vi "2BALL1~1.VI"(1 "Run?":bool) -> (0 "Done?":bool)   [LabVIEW 2013]
uses:
  Globals/Homes.vi
  Globals/Useful Values.vi
panel:
  out "Time Elapsed":dbl
  out "Sum":dbl
  out "Ready for Vision?":bool
  out "Side":dbl
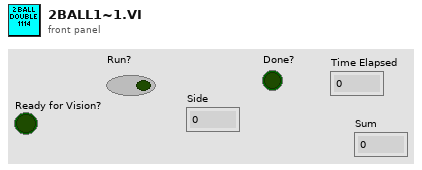
[diagram p1: front panel]
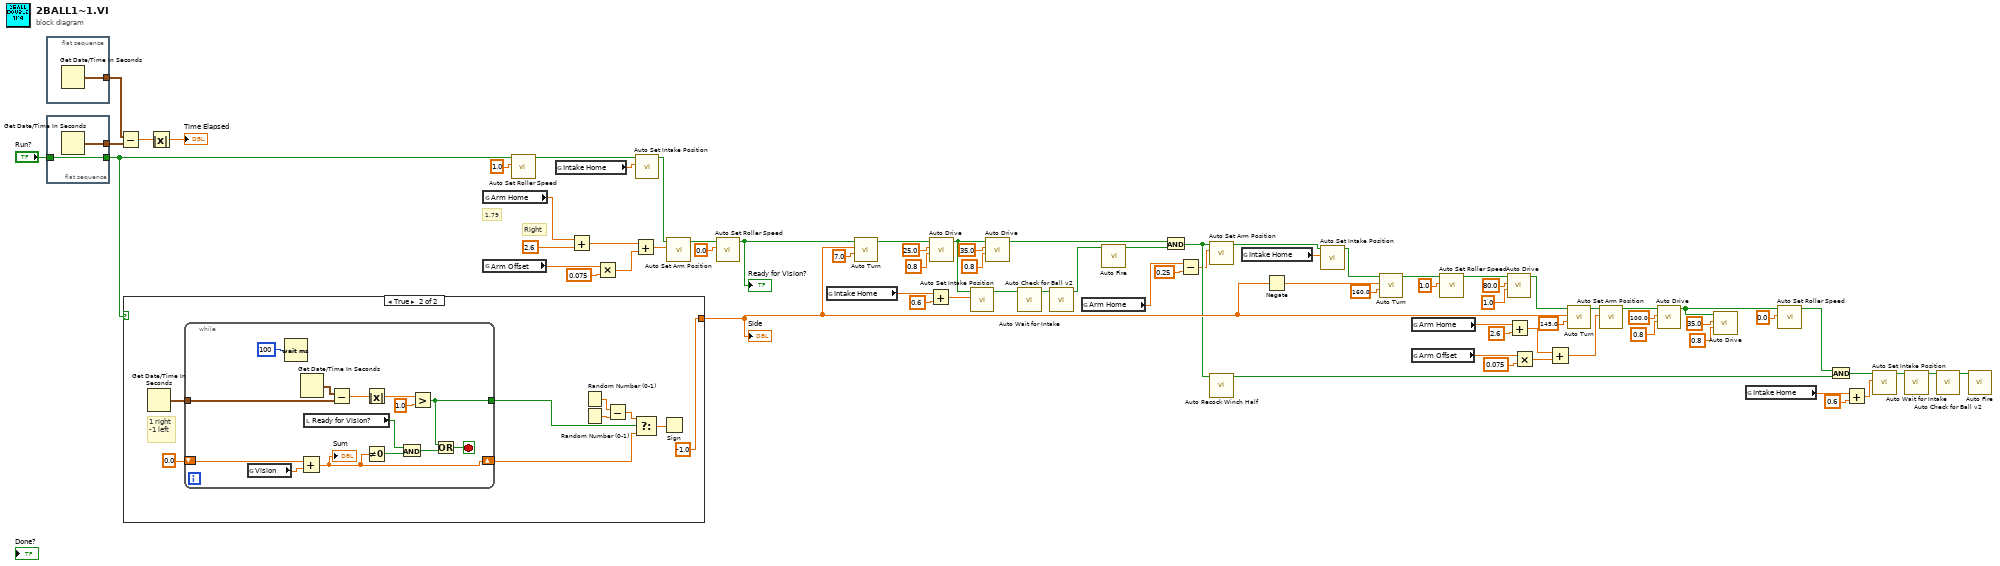
[diagram p0: block diagram]
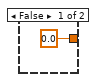
[diagram p2: hidden frame]
diagram:
  # "Right"
  # "1.79"
  n1 = flat-sequence {
    tunnel: [w77] -> w64
    frame #0 {
      n2 = Get Date/Time In Seconds() -> (seconds since 1Jan1904=w77:timestamp)
    }
  }
  n3 = flat-sequence {
    tunnel: "Run?" -> [w79]
    tunnel: [w79] -> w65
    tunnel: [w78] -> w61
    frame #0 {
      n4 = Get Date/Time In Seconds() -> (seconds since 1Jan1904=w78:timestamp)
    }
  }
  n5 = Subtract(x=w64, y=w61) -> (x-y=w63:dbl)
  n6 = case shown="True" w65 {
    tunnel: [0.0 -1.0] -> w56
    frame False {
    }
    frame True {
      # "1 right\n-1 left"
      n7 = Get Date/Time In Seconds() -> (seconds since 1Jan1904=w88:timestamp)
      n8 = while {
        shift-right: [w99] -> w83
        shift-left: 0.0 -> [w102]
        tunnel: w88 -> [w97]
        tunnel: [w90] -> w84
        stop <- w92 stop-if-true
        n9 = global read "Useful Values.vi" "Vision"() -> (w103:dbl)
        n10 = Wait (ms)(milliseconds to wait=u32 100) -> ()  [unwired: 1 out]
        n11 = Add(x=w102, y=w103) -> (x+y=w99:dbl)
        "Sum" <- w99
        n12 = Get Date/Time In Seconds() -> (seconds since 1Jan1904=w96:timestamp)
        n13 = local read "Ready for Vision?"() -> (w100:bool)
        n14 = Subtract(x=w96, y=w97) -> (x-y=w95:dbl)
        n15 = Absolute Value(x=w95) -> (abs(x)=w94:dbl)
        n16 = Not Equal To 0?(x=w99) -> (x != 0?=w98:bool)
        n17 = And(x=w100, y=w98) -> (x .and. y?=w91:bool)
        n18 = Greater?(x=w94, y=1.0) -> (0:w90:bool)
        n19 = Or(x=w90, y=w91) -> (x .or. y?=w92:bool)
      }
      n20 = Random Number (0-1)() -> (number: 0 to 1=w85:dbl)
      n21 = Random Number (0-1)() -> (number: 0 to 1=w86:dbl)
      n22 = Subtract(x=w85, y=w86) -> (x-y=w87:dbl)
      n23 = Select(t=w87, s=w84, f=w83) -> (s? t:f=w82:dbl)
      n24 = Sign(1:w82) -> ()  [unwired: 1 out]
    }
  }
  "Side" <- w56
  n25 = Absolute Value(x=w63) -> (abs(x)=→"Time Elapsed":dbl)
  n26 = global read "Homes.vi" "Arm Home"() -> (w75:dbl)
  n27 = global read "Useful Values.vi" "Arm Offset"() -> (w73:dbl)
  n28 = call "Auto Set Roller Speed.vi"("Value"=1.0, "Run?"=w65) -> ("Done"=w68:bool)  [unwired: 9 in]
  n29 = global read "Homes.vi" "Intake Home"() -> (w76:dbl)
  n30 = Add(x=w75, y=2.6) -> (x+y=w70:dbl)
  n31 = Multiply(x=w73, y=0.075) -> (x*y=w71:dbl)
  n32 = Add(x=w70, y=w71) -> (x+y=w59:dbl)
  n33 = call "Auto Set Intake Position.vi"("Intake Position"=w76, "Run?"=w68) -> ("Done"=w60:bool)  [unwired: 9 in]
  n34 = call "Auto Set Arm Position.vi"("Arm Position"=w59, "Run?"=w60) -> ("Done"=w58:bool)  [unwired: 9 in]
  n35 = call "Auto Set Roller Speed.vi"("Value"=0.0, "Run?"=w58) -> ("Done"=w57:bool)  [unwired: 9 in]
  "Ready for Vision?" <- w57
  n36 = global read "Homes.vi" "Intake Home"() -> (w50:dbl)
  n37 = call "Auto Turn.vi"("Turn Amount"=7.0, "+/-?"=w56, "Run?"=w57) -> ("Done"=w47:bool)  [unwired: 8 in]
  n38 = Add(x=w50, y=0.6) -> (x+y=w48:dbl)
  n39 = call "Auto Drive.vi"("Speed"=0.8, "Amount"=25.0, "Run?"=w47) -> ("Done"=w41:bool)  [unwired: 8 in]
  n40 = call "Auto Set Intake Position.vi"("Intake Position"=w48, "Run?"=w41) -> ("Done"=w46:bool)  [unwired: 9 in]
  n41 = call "Auto Drive.vi"("Speed"=0.8, "Amount"=35.0, "Run?"=w41) -> ("Done"=w44:bool)  [unwired: 8 in]
  n42 = call "Auto Wait for Intake.vi"("Run?"=w46) -> ("Done"=w43:bool)  [unwired: 10 in]
  n43 = call "Auto Check for Ball v2.vi"("Run?"=w43) -> ("Done"=w42:bool)  [unwired: 10 in]
  n44 = global read "Homes.vi" "Arm Home"() -> (w34:dbl)
  n45 = call "Auto Fire.vi"("Run?"=w42) -> ("Done"=w45:bool)  [unwired: 10 in]
  n46 = And(x=w44, y=w45) -> (x .and. y?=w35:bool)
  n47 = Subtract(x=w34, y=0.25) -> (x-y=w32:dbl)
  n48 = call "Auto Set Arm Position.vi"("Arm Position"=w32, "Run?"=w35) -> ("Done"=w31:bool)  [unwired: 9 in]
  n49 = call "Auto Recock Winch Half.vi"("Run?"=w35) -> ("Done"=w12:bool)  [unwired: 10 in]
  n50 = global read "Homes.vi" "Intake Home"() -> (w29:dbl)
  n51 = Negate(x=w56) -> (-x=w5:dbl)
  n52 = call "Auto Set Intake Position.vi"("Intake Position"=w29, "Run?"=w31) -> ("Done"=w30:bool)  [unwired: 9 in]
  n53 = call "Auto Turn.vi"("Turn Amount"=160.0, "+/-?"=w5, "Run?"=w30) -> ("Done"=w37:bool)  [unwired: 8 in]
  n54 = global read "Homes.vi" "Arm Home"() -> (w21:dbl)
  n55 = global read "Useful Values.vi" "Arm Offset"() -> (w25:dbl)
  n56 = call "Auto Set Roller Speed.vi"("Value"=1.0, "Run?"=w37) -> ("Done"=w38:bool)  [unwired: 9 in]
  n57 = call "Auto Drive.vi"("Speed"=1.0, "Amount"=80.0, "Run?"=w38) -> ("Done"=w19:bool)  [unwired: 8 in]
  n58 = Add(x=w21, y=2.6) -> (x+y=w22:dbl)
  n59 = Multiply(x=w25, y=0.075) -> (x*y=w23:dbl)
  n60 = Add(x=w22, y=w23) -> (x+y=w20:dbl)
  n61 = call "Auto Turn.vi"("Turn Amount"=145.0, "+/-?"=w56, "Run?"=w19) -> ("Done"=w18:bool)  [unwired: 8 in]
  n62 = call "Auto Set Arm Position.vi"("Arm Position"=w20, "Run?"=w18) -> ("Done"=w1:bool)  [unwired: 9 in]
  n63 = call "Auto Drive.vi"("Speed"=0.8, "Amount"=100.0, "Run?"=w1) -> ("Done"=w3:bool)  [unwired: 8 in]
  n64 = call "Auto Drive.vi"("Speed"=0.8, "Amount"=35.0, "Run?"=w3) -> ()  [unwired: 8 in, 1 out]
  n65 = global read "Homes.vi" "Intake Home"() -> (w8:dbl)
  n66 = call "Auto Set Roller Speed.vi"("Value"=0.0, "Run?"=w3) -> ("Done"=w2:bool)  [unwired: 9 in]
  n67 = And(x=w2, y=w12) -> (x .and. y?=w7:bool)
  n68 = Add(x=w8, y=0.6) -> (x+y=w10:dbl)
  n69 = call "Auto Set Intake Position.vi"("Intake Position"=w10, "Run?"=w7) -> ("Done"=w11:bool)  [unwired: 9 in]
  n70 = call "Auto Wait for Intake.vi"("Run?"=w11) -> ("Done"=w6:bool)  [unwired: 10 in]
  n71 = call "Auto Check for Ball v2.vi"("Run?"=w6) -> ("Done"=w13:bool)  [unwired: 10 in]
  n72 = call "Auto Fire.vi"("Run?"=w13) -> ()  [unwired: 10 in, 1 out]
